vi "Strip Symmetric.vi"(3 "String":string, 4 "Num Chars (1)":i32=1) -> (5 "String":string)   [LabVIEW 2014, in "LMH-Toolbox.lvlib"]
doc: "Strip the specified number of characters from each end of the specified string. This VI is useful for removeing quotes, brackets, etc."
uses:
  <vilib>/MakerHub/Toolbox/LMH-Toolbox.lvlib
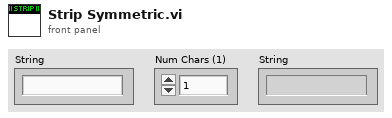
[diagram p1: front panel]
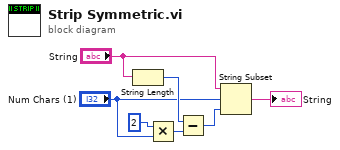
[diagram p0: block diagram]
diagram:
  n1 = String Length(string="String") -> (length=w7:i32)
  n2 = Multiply(x=2 ("y"), y="Num Chars (1)") -> (x*y=w1:i32)
  n3 = Subtract(x=w7, y=w1) -> (x-y=w6:i32)
  n4 = String Subset(string="String", offset (0)="Num Chars (1)", length (rest)=w6) -> (substring=→"String":string)
